vi "LVCAM Create Nest.vi"(9 "Nest Alias":string, 10 "Nest Actor":refnum<class "LVCAM.lvclass">, 11 "Actor in":refnum<class "Actor.lvclass">) -> (0 "error out":errorcluster, 3 "Actor out":refnum<class "Actor.lvclass">)   [LabVIEW 2021, in "LVCAM.lvlib" / "Actor.lvclass"]
uses:
  Actor.lvclass
  C:/PPLs/LabVIEW-Composed-Actor-Model-LVCAM/LabVIEW-Composed-Actor-Model-LVCAM/LVCAM/LVCAM/LVCAM/LVCAM.lvclass
  LVCAM/LVCAM.lvclass
  Actor.lvclass/Actor.ctl
  LVCAM/Msg Loop.vi
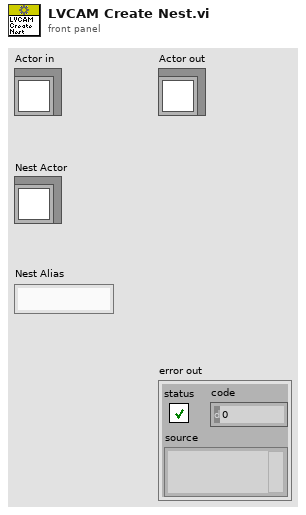
[diagram p1: front panel]
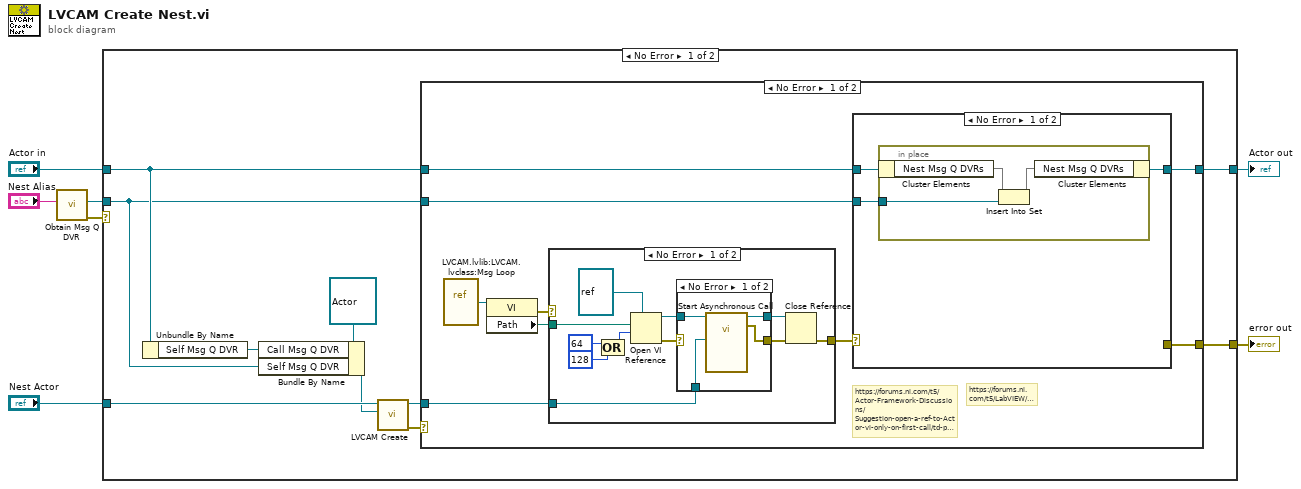
[diagram p0: block diagram]
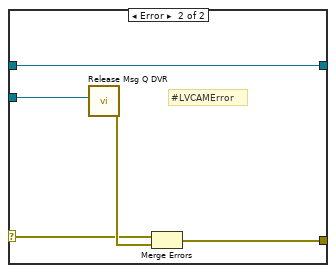
[diagram p4: hidden frame]
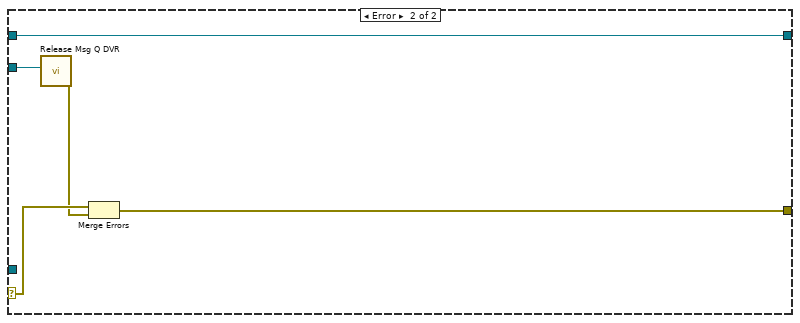
[diagram p5: hidden frame]
diagram:
  n1 = call "Obtain Msg Q DVR.vi"("Msg Q DVR Alias"="Nest Alias") -> ("error out"=w1:errorcluster, "Msg Q DVR"=w3:refnum<data-value>)  [unwired: 9 in]
  n2 = case shown="No Error" w1 {
    selector: w1 -> [_ w62]
    tunnel: [w17 w61] -> w7
    tunnel: [w15 w62] -> w4
    tunnel: "Nest Actor" -> [w13 _]
    tunnel: w3 -> [w10 _]
    tunnel: "Actor in" -> [w12 w61]
    frame No Error {
      n3 = Unbundle By Name(w12) -> ("Self Msg Q DVR"=w11:refnum<data-value>)
      n4 = Bundle By Name(cluster=refnum<class "Actor.lvclass"> refnum ("Self Actor in"), "Call Msg Q DVR"=w11, "Self Msg Q DVR"=w10) -> (w9:refnum<class "Actor.lvclass">)
      n5 = call-dynamic "LVCAM Create.vi"("Actor"=w9, "LVCAM Create in"=w13) -> ("error out"=w8:errorcluster, "LVCAM Create out"=w16:refnum<class "LVCAM.lvclass">)  [unwired: 8 in]
      n6 = case shown="No Error" w8 {
        selector: w8 -> [_ w60]
        tunnel: [w26 w58] -> w17
        tunnel: w16 -> [w25 _]
        tunnel: [w24 w57] -> w15
        tunnel: w12 -> [w22 w58]
        tunnel: w10 -> [w21 w59]
        frame No Error {
          # "https://forums.ni.com/t5/LabVIEW/Static-VI-Reference/m-p/3334014#M978333"
          # "https://forums.ni.com/t5/Actor-Framework-Discussions/Suggestion-open-a-ref-to-Actor-vi-only-on-first-call/td-p/3451643/page/4"
          n7 = vi-ref "LVCAM.lvlib:LVCAM.lvclass:Msg Loop.vi"() -> (w19:refnum<vi>)
          n8 = property class="VI"(reference=w19) -> (error out=w20:errorcluster, "Path"=w18:path)  [unwired: 1 in, 1 out]
          n9 = case shown="No Error" w20 {
            selector: w20 -> [_ w44]
            tunnel: [w35 w44] -> w23
            tunnel: w18 -> [w31 _]
            tunnel: w25 -> [w27 _]
            frame No Error {
              n10 = Compound Arithmetic op=OR(64 ("options: Multiple Clones,\n  Fire & Forget"), 128 ("options: Multiple Clones,\n  Fire & Forget")) -> (w33:i32)
              n11 = Open VI Reference(type specifier VI Refnum (for type only)=refnum<vi> refnum, vi path=w31, options=w33) -> (vi reference=w29:refnum<vi>, error out=w30:errorcluster)  [unwired: 3 in]
              n12 = case shown="No Error" w30 {
                selector: w30 -> [_ w43]
                tunnel: [w41 w42] -> w37
                tunnel: [w40 w43] -> w36
                tunnel: w29 -> [w39 w42]
                tunnel: w27 -> [w38 _]
                frame No Error {
                  n13 = call-by-ref "Start Asynchronous Call"(reference=w39, "LVCAM in"=w38) -> (reference out=w41:refnum<vi>, error out=w40:errorcluster)  [unwired: 12 in]
                }
                frame Error {
                }
              }
              n14 = Close Reference(reference=w37, error in (no error)=w36) -> (error out=w35:errorcluster)
            }
            frame Error {
            }
          }
          n15 = case shown="No Error" w23 {
            selector: w23 -> [_ w51]
            tunnel: w22 -> [w47 w55]
            tunnel: [w46 w55] -> w26
            tunnel: w21 -> [w45 w54]
            tunnel: [_ w53] -> w24
            frame No Error {
              n16 = in-place {
                in-place-border: w45 -> [w48]
                n17 = in-place-cluster #1(w47) -> ("Nest Msg Q DVRs"=w50:set{refnum<data-value>})
                n18 = Insert Into Set(10:w48, 11:w50) -> (3:w49:set{refnum<data-value>})  [unwired: 1 out]
                n19 = in-place-cluster #1("Nest Msg Q DVRs"=w49) -> (w46:refnum<class "Actor.lvclass">)
              }
            }
            frame Error {
              # "#LVCAMError"
              n20 = call "Release Msg Q DVR.vi"("Msg Q DVR"=w54) -> ("error out"=w52:errorcluster)  [unwired: 10 in]
              n21 = Merge Errors(w51, w52) -> (w53:errorcluster)
            }
          }
        }
        frame Error {
          n22 = call "Release Msg Q DVR.vi"("Msg Q DVR"=w59) -> ("error out"=w56:errorcluster)  [unwired: 10 in]
          n23 = Merge Errors(w60, w56) -> (w57:errorcluster)
        }
      }
    }
    frame Error {
      # "#LVCAMError"
    }
  }
  "error out" <- w4
  "Actor out" <- w7
